vi "CAN Task.vi"(8 "error in":errorcluster, 11 "CANopen Master in":refnum<class "CANopen Master.lvclass">) -> ()   [LabVIEW 2024, in "CANopen Master.lvclass"]
uses:
  CANopen Master.lvclass
  CANopen Master.lvclass/CANopen Master.ctl
  CANopen Response/CANopen Response Message.lvclass
  source/CANopen Message/CANopen Message.lvclass
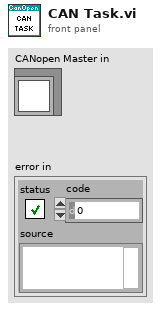
[diagram p1: front panel]
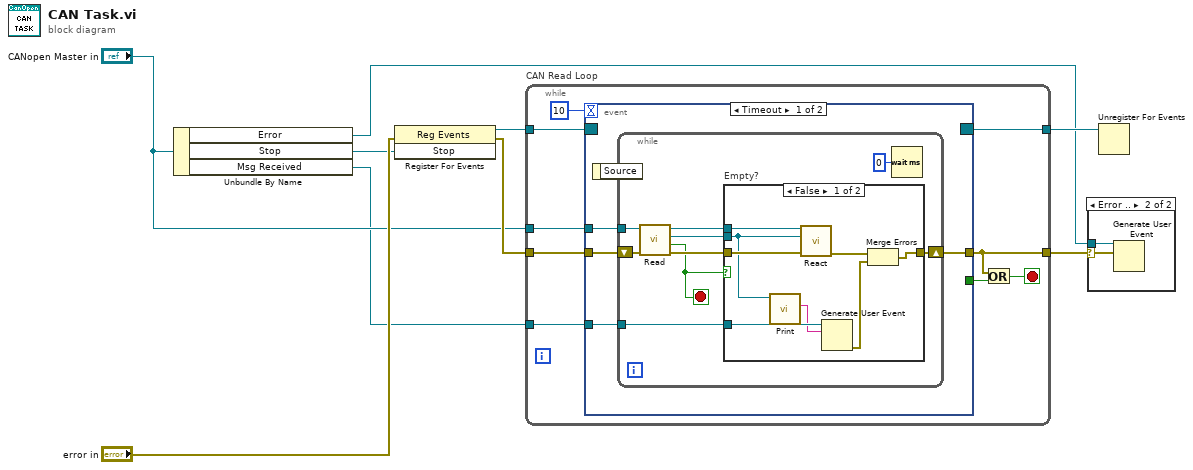
[diagram p0: block diagram]
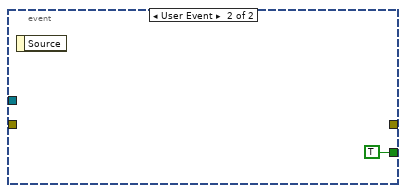
[diagram p4: hidden frame]
diagram:
  n1 = Unbundle By Name("CANopen Master in") -> ("Error"=w1:refnum<user-event>, "Stop"=w3:refnum<user-event>, "Msg Received"=w2:refnum<user-event>)
  n2 = register-events(error in="error in", w3) -> (reference out=w4:refnum<event-registration>, error out=w8:errorcluster)  [unwired: 1 in]
  n3 = while "CAN Read Loop" {
    tunnel: [w13] -> w6
    tunnel: w4 -> [w12]
    tunnel: w2 -> [w10]
    tunnel: "CANopen Master in" -> [w16]
    tunnel: w8 -> [w18]
    tunnel: [w17] -> w7
    stop <- w15 stop-if-true
    n4 = event shown="[0] Timeout" {
      selector: w12 -> [_ _]
      dyn-events: [_ _] -> w13
      timeout: 10 -> [_ _]
      tunnel: w18 -> [w22 _]
      tunnel: w16 -> [w20 _]
      tunnel: [w21 _] -> w17
      tunnel: [_ TRUE] -> w11
      tunnel: w10 -> [w19 _]
      event Timeout {
        n5 = event-data() -> ()  [unwired: 1 in, 1 out]
        n6 = while {
          tunnel: w20 -> [w28]
          tunnel: w19 -> [w27]
          shift-right: [w30] -> w21
          shift-left: w22 -> [w31]
          stop <- w23 stop-if-true
          n7 = call "Read.vi"("error in"=w31, "CANopen Master in"=w28) -> ("error out"=w29:errorcluster, "Empty?"=w23:bool, "CANopen Message out"=w26:refnum<class "CANopen Response Message.lvclass">, "CANopen Master out"=w24:refnum<class "CANopen Master.lvclass">)  [unwired: 6 in]
          n8 = case "Empty?" shown="False" w23 {
            tunnel: w26 -> [w34 _]
            tunnel: [w37 w40] -> w30
            tunnel: w29 -> [w39 w40]
            tunnel: w24 -> [w35 _]
            tunnel: w27 -> [w33 _]
            frame False {
              n9 = call "Print.vi"("CANopen Message in"=w34) -> ("Message"=w32:string)  [unwired: 9 in, 1 out]
              n10 = call "React.vi"("error in"=w39, "CANopen Message"=w34, "CANopen Master in"=w35) -> ("error out"=w38:errorcluster)  [unwired: 7 in, 1 out]
              n11 = Generate User Event(user event=w33, event data cluster=w32) -> (error out=w36:errorcluster)  [unwired: 2 in, 1 out]
              n12 = Merge Errors(w38, w36) -> (w37:errorcluster)
            }
            frame True {
            }
          }
          n13 = Wait (ms)(milliseconds to wait=u32 0) -> ()  [unwired: 1 out]
        }
      }
      event User Event {
        n14 = event-data() -> ()  [unwired: 1 in, 1 out]
      }
    }
    n15 = Or(x=w17, y=w11) -> (x .or. y?=w15:bool)
  }
  n16 = case shown="Error .." w7 {
    selector: w7 -> [_ w43]
    tunnel: w1 -> [_ w42]
    frame No Error {
    }
    frame Error {
      n17 = Generate User Event(user event=w42, event data cluster=w43) -> ()  [unwired: 2 in, 2 out]
    }
  }
  n18 = Unregister For Events(event registration refnum=w6) -> ()  [unwired: 1 in, 1 out]
